vi "Main.vi"   [LabVIEW 2020]
uses:
  Controls/Application Event Message.ctl
  Controls/Application Events.ctl
  Controls/Application Modules.ctl
  Controls/Module Message.ctl
  Error/Controls/Error Message.ctl
  Controls/Module Operational Loop Data.ctl
  Controls/Module State.ctl
types:
  T1 = typedef "Application Events.ctl" = enum16{"Initialize", "Shutdown", "UI: Login", "UI: Withdrawal", "UI: Terminate", "UI: Fast Cash", "UI: Balance Inquiry", "UI: Deposit", "UI: New Transaction", "UI: Card Reader", "UI: On Account Number", "UI: Transaction Timeout", "Controller: Idle", "Controller: Invalid Login", "Controller: Broadcast Balance "}
  T2 = typedef "Module State.ctl" = enum16{"Initial", "Idle", "Login", "Balance Inquiry", "Deposit", "Withdrawal", "Fast Cash", "Terminate"}
  T3 = typedef "Module Operational Loop Data.ctl" = cluster{"State":T2}
  T4 = typedef "Error Message.ctl" = cluster{"Source":T5, "Event":T1, "Error To Handle":errorcluster}
  T5 = typedef "Application Modules.ctl" = enum16{"Controller", "User Console", "Display Console", "Error Handler", "Database Module"}
  T6 = typedef "Module Message.ctl" = cluster{"Source":T5, "Event":T1, "Data":variant}
  T7 = typedef "Application Event Message.ctl" = cluster{"Source":T5, "Event":T1, "Data":variant}
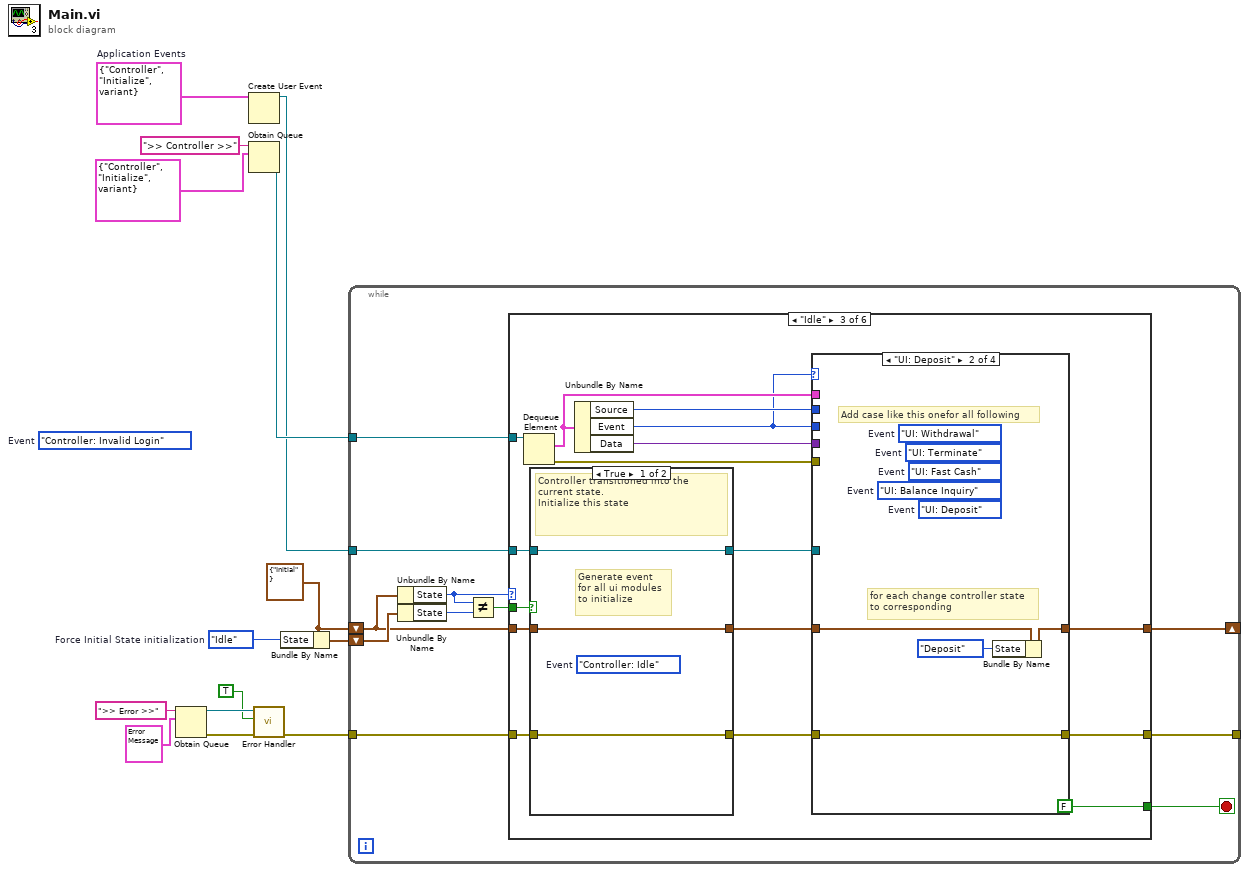
[diagram p0: block diagram]
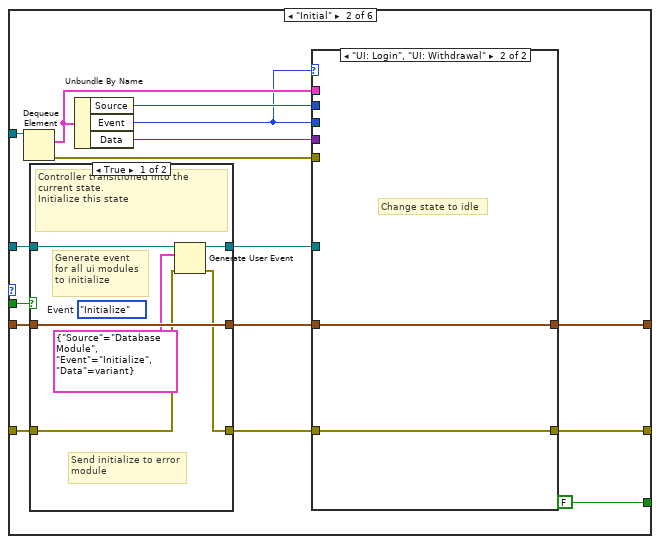
[diagram p3: hidden frame]
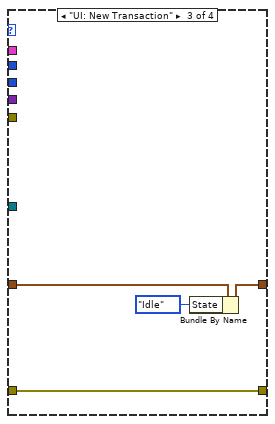
[diagram p7: hidden frame]
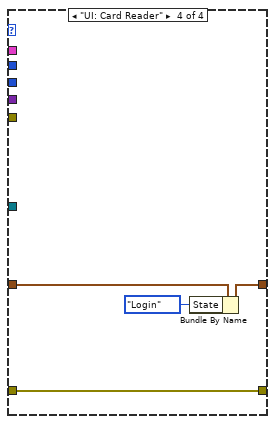
[diagram p8: hidden frame]
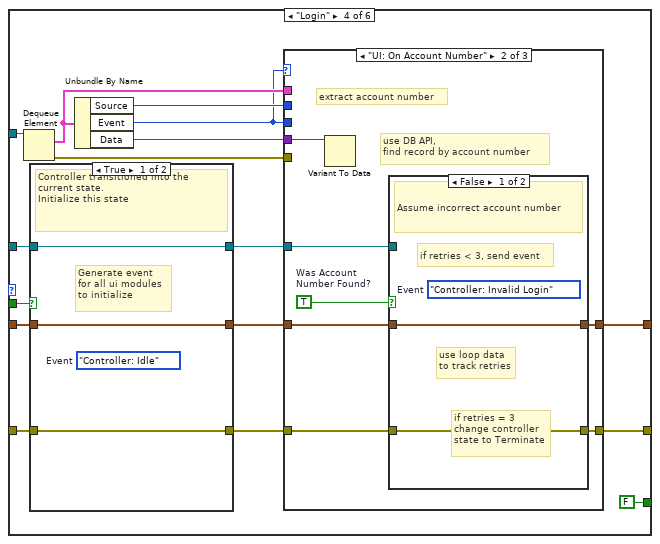
[diagram p10: hidden frame]
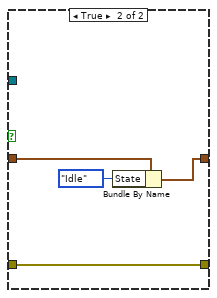
[diagram p12: hidden frame]
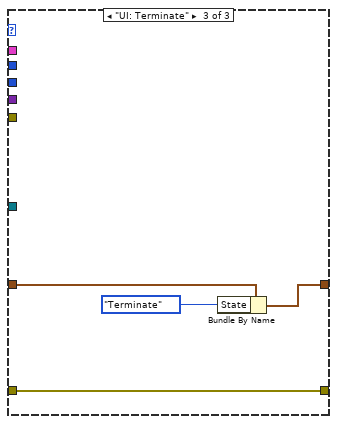
[diagram p13: hidden frame]
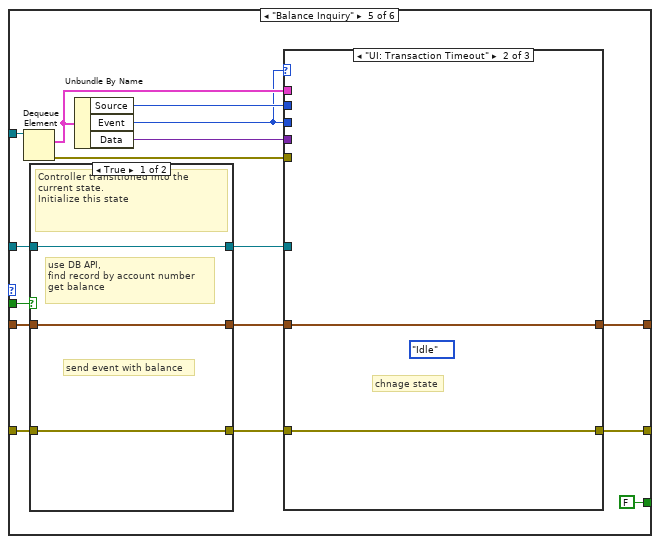
[diagram p15: hidden frame]
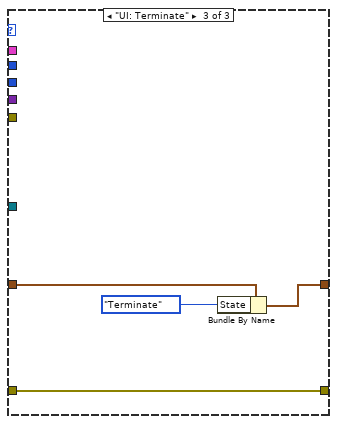
[diagram p17: hidden frame]
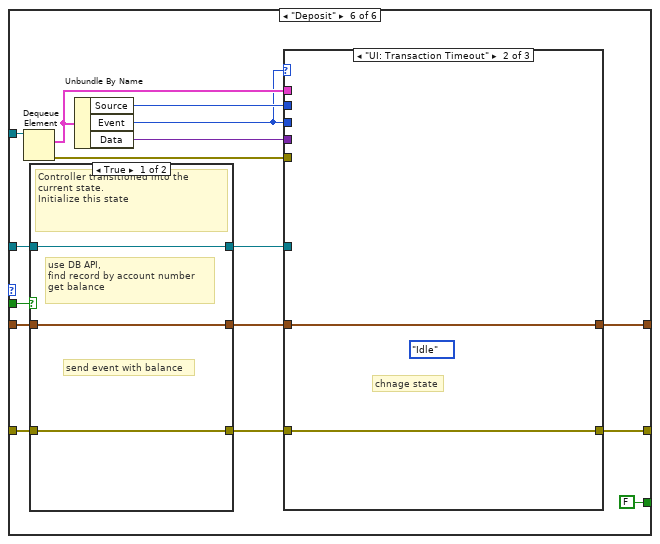
[diagram p19: hidden frame]
diagram:
  (unwired) Application_Events."Controller: Invalid Login"  # Event
  w1 = Module_State."Idle"  # Force Initial State initialization
  w3 = T3 {"State"=enum."Initial"}
  w14 = T7 {"Source"=enum."Controller", "Event"=enum."Initialize", "Data"=variant}  # Application Events
  n1 = Obtain Queue(name (unnamed)=">> Error >>", element data type=T4 {"Source"=enum."Controller", "Event"=enum."Initialize", "Error To Handle"={"status"=FALSE, "code"=0, "source"=""}}) -> (queue out=w8:refnum<queue>, error out=w9:errorcluster)  [unwired: 3 in, 1 out]
  n2 = Create User Event(user event datatype=w14) -> (user event=w4:refnum<user-event>)  [unwired: 1 in, 1 out]
  n3 = Obtain Queue(name (unnamed)=">> Controller >>", element data type=T6 {"Source"=enum."Controller", "Event"=enum."Initialize", "Data"=variant}) -> (queue out=w5:refnum<queue>)  [unwired: 3 in, 2 out]
  n4 = call "Error Handler.vi"("error in"=w9, "Load Reference?"=TRUE, "Error Queue"=w8) -> ("error out"=w6:errorcluster)  [unwired: 8 in]
  n5 = Bundle By Name(cluster=w3, "State"=w1) -> (w2:T3)
  n6 = while {
    tunnel: w6 -> [w17]
    shift-right: [w25] -> _
    shift-left: w3 -> [w23]
    shift-left: w2 -> [w24]
    tunnel: w5 -> [w18]
    tunnel: [w16] -> _
    tunnel: w4 -> [w15]
    stop <- w20 stop-if-true
    n7 = Unbundle By Name(w23) -> ("State"=w21:T2)
    n8 = Unbundle By Name(w24) -> ("State"=w22:T2)
    n9 = Not Equal?(x=w21, y=w22) -> (x != y?=w19:bool)
    n10 = case shown="\"Idle\"" w21 {
      tunnel: [w27 w36 w65 w101 w142 w172] -> w25
      tunnel: w23 -> [w27 w42 w71 w107 w148 w178]
      tunnel: [_ FALSE FALSE FALSE FALSE FALSE] -> w20
      tunnel: w19 -> [_ w41 w70 w106 w147 w177]
      tunnel: w18 -> [_ w40 w69 w105 w146 w176]
      tunnel: [w26 w38 w67 w103 w144 w174] -> w16
      tunnel: w17 -> [w26 w39 w68 w104 w145 w175]
      tunnel: w15 -> [_ w28 w57 w93 w134 w164]
      frame Default {
      }
      frame "Initial" {
        n11 = Dequeue Element(queue=w40) -> (element=w34:T6, error out=w30:errorcluster)  [unwired: 2 in, 2 out]
        n12 = case shown="True" w41 {
          tunnel: [w53 w56] -> w35
          tunnel: w42 -> [w53 w56]
          tunnel: [w50 w55] -> w37
          tunnel: w39 -> [w51 w55]
          tunnel: [w49 w54] -> w29
          tunnel: w28 -> [w52 w54]
          frame True {
            (unwired) Application_Events."Initialize"  # Event
            # "Send initialize to error\nmodule"
            # "Generate event\nfor all ui modules\nto initialize"
            # "Controller transitioned into the current state.\nInitialize this state"
            n13 = Generate User Event(user event=w52, event data cluster=T7 {"Source"=enum."Database Module", "Event"=enum."Initialize", "Data"=variant} ("event data"), error in=w51) -> (user event out=w49:refnum<user-event>, error out=w50:errorcluster)  [unwired: 1 in]
          }
          frame False {
            # "No State transisiton detected"
          }
        }
        n14 = Unbundle By Name(w34) -> ("Source"=w33:T5, "Event"=w31:T1, "Data"=w32:variant)
        n15 = case shown="\"UI: Login\", \"UI: Withdrawal\"" w31 {
          tunnel: [w45 w47] -> w38
          tunnel: w37 -> [w45 w47]
          tunnel: [w44 w46] -> w36
          tunnel: w35 -> [w44 w46]
          tunnel: w34 -> [_ _]
          tunnel: w33 -> [_ _]
          tunnel: w31 -> [_ _]
          tunnel: w32 -> [_ _]
          tunnel: w30 -> [_ _]
          tunnel: w29 -> [_ _]
          frame Default {
          }
          frame "UI: Login", "UI: Withdrawal" {
            # "Change state to idle"
          }
        }
      }
      frame "Idle" {
        n16 = Dequeue Element(queue=w69) -> (element=w63:T6, error out=w59:errorcluster)  [unwired: 2 in, 2 out]
        n17 = case shown="True" w70 {
          tunnel: [w89 w92] -> w64
          tunnel: w71 -> [w89 w92]
          tunnel: [w88 w91] -> w66
          tunnel: w68 -> [w88 w91]
          tunnel: [w87 w90] -> w58
          tunnel: w57 -> [w87 w90]
          frame True {
            (unwired) Application_Events."Controller: Idle"  # Event
            # "Generate event\nfor all ui modules\nto initialize"
            # "Controller transitioned into the current state.\nInitialize this state"
          }
          frame False {
            # "No State transisiton detected"
          }
        }
        n18 = Unbundle By Name(w63) -> ("Source"=w62:T5, "Event"=w60:T1, "Data"=w61:variant)
        n19 = case shown="\"UI: Deposit\"" w60 {
          tunnel: [w74 w78 w82 w86] -> w67
          tunnel: w66 -> [w74 w78 w82 w86]
          tunnel: [w73 w75 w79 w83] -> w65
          tunnel: w64 -> [w73 w77 w81 w85]
          tunnel: w63 -> [_ _ _ _]
          tunnel: w62 -> [_ _ _ _]
          tunnel: w60 -> [_ _ _ _]
          tunnel: w61 -> [_ _ _ _]
          tunnel: w59 -> [_ _ _ _]
          tunnel: w58 -> [_ _ _ _]
          frame Default {
          }
          frame "UI: Deposit" {
            (unwired) Application_Events."UI: Deposit"  # Event
            (unwired) Application_Events."UI: Balance Inquiry"  # Event
            (unwired) Application_Events."UI: Fast Cash"  # Event
            (unwired) Application_Events."UI: Terminate"  # Event
            (unwired) Application_Events."UI: Withdrawal"  # Event
            # "for each change controller state\nto corresponding"
            # "Add case like this onefor all following"
            n20 = Bundle By Name(cluster=w77, "State"=Module_State."Deposit") -> (w75:T3)
          }
          frame "UI: New Transaction" {
            n21 = Bundle By Name(cluster=w81, "State"=Module_State."Idle") -> (w79:T3)
          }
          frame "UI: Card Reader" {
            n22 = Bundle By Name(cluster=w85, "State"=Module_State."Login") -> (w83:T3)
          }
        }
      }
      frame "Login" {
        n23 = Dequeue Element(queue=w105) -> (element=w99:T6, error out=w95:errorcluster)  [unwired: 2 in, 2 out]
        n24 = case shown="True" w106 {
          tunnel: [w130 w133] -> w100
          tunnel: w107 -> [w130 w133]
          tunnel: [w129 w132] -> w102
          tunnel: w104 -> [w129 w132]
          tunnel: [w128 w131] -> w94
          tunnel: w93 -> [w128 w131]
          frame True {
            (unwired) Application_Events."Controller: Idle"  # Event
            # "Generate event\nfor all ui modules\nto initialize"
            # "Controller transitioned into the current state.\nInitialize this state"
          }
          frame False {
            # "No State transisiton detected"
          }
        }
        n25 = Unbundle By Name(w99) -> ("Source"=w98:T5, "Event"=w96:T1, "Data"=w97:variant)
        n26 = case shown="\"UI: On Account Number\"" w96 {
          tunnel: [w110 w113 w127] -> w103
          tunnel: w102 -> [w110 w112 w127]
          tunnel: [w109 w116 w124] -> w101
          tunnel: w100 -> [w109 w117 w126]
          tunnel: w99 -> [_ _ _]
          tunnel: w98 -> [_ _ _]
          tunnel: w96 -> [_ _ _]
          tunnel: w97 -> [_ w115 _]
          tunnel: w95 -> [_ _ _]
          tunnel: w94 -> [_ w111 _]
          frame Default {
          }
          frame "UI: On Account Number" {
            w114 = TRUE  # Was Account  Number Found?
            # "use DB API,\nfind record by account number"
            # "extract account number"
            n27 = Variant To Data(Variant=w115) -> ()  [unwired: 2 in, 2 out]
            n28 = case shown="False" w114 {
              tunnel: w117 -> [w119 w123]
              tunnel: [w119 w121] -> w116
              tunnel: [w118 w120] -> w113
              tunnel: w112 -> [w118 w120]
              tunnel: w111 -> [_ _]
              frame False {
                (unwired) Application_Events."Controller: Invalid Login"  # Event
                # "if retries < 3, send event"
                # "if retries = 3\nchange controller\nstate to Terminate"
                # "use loop data\nto track retries"
                # "Assume incorrect account number"
              }
              frame True {
                n29 = Bundle By Name(cluster=w123, "State"=Module_State."Idle") -> (w121:T3)
              }
            }
          }
          frame "UI: Terminate" {
            n30 = Bundle By Name(cluster=w126, "State"=Module_State."Terminate") -> (w124:T3)
          }
        }
      }
      frame "Balance Inquiry" {
        n31 = Dequeue Element(queue=w146) -> (element=w140:T6, error out=w136:errorcluster)  [unwired: 2 in, 2 out]
        n32 = case shown="True" w147 {
          tunnel: [w160 w163] -> w141
          tunnel: w148 -> [w160 w163]
          tunnel: [w159 w162] -> w143
          tunnel: w145 -> [w159 w162]
          tunnel: [w158 w161] -> w135
          tunnel: w134 -> [w158 w161]
          frame True {
            # "send event with balance"
            # "use DB API,\nfind record by account number\nget balance"
            # "Controller transitioned into the current state.\nInitialize this state"
          }
          frame False {
            # "No State transisiton detected"
          }
        }
        n33 = Unbundle By Name(w140) -> ("Source"=w139:T5, "Event"=w137:T1, "Data"=w138:variant)
        n34 = case shown="\"UI: Transaction Timeout\"" w137 {
          tunnel: [w151 w152 w157] -> w144
          tunnel: w143 -> [w151 w152 w157]
          tunnel: [w150 w153 w154] -> w142
          tunnel: w141 -> [w150 w153 w156]
          tunnel: w140 -> [_ _ _]
          tunnel: w139 -> [_ _ _]
          tunnel: w137 -> [_ _ _]
          tunnel: w138 -> [_ _ _]
          tunnel: w136 -> [_ _ _]
          tunnel: w135 -> [_ _ _]
          frame Default {
          }
          frame "UI: Transaction Timeout" {
            (unwired) Module_State."Idle" ("State")
            # "chnage state"
          }
          frame "UI: Terminate" {
            n35 = Bundle By Name(cluster=w156, "State"=Module_State."Terminate") -> (w154:T3)
          }
        }
      }
      frame "Deposit" {
        n36 = Dequeue Element(queue=w176) -> (element=w170:T6, error out=w166:errorcluster)  [unwired: 2 in, 2 out]
        n37 = case shown="True" w177 {
          tunnel: [w190 w193] -> w171
          tunnel: w178 -> [w190 w193]
          tunnel: [w189 w192] -> w173
          tunnel: w175 -> [w189 w192]
          tunnel: [w188 w191] -> w165
          tunnel: w164 -> [w188 w191]
          frame True {
            # "send event with balance"
            # "use DB API,\nfind record by account number\nget balance"
            # "Controller transitioned into the current state.\nInitialize this state"
          }
          frame False {
            # "No State transisiton detected"
          }
        }
        n38 = Unbundle By Name(w170) -> ("Source"=w169:T5, "Event"=w167:T1, "Data"=w168:variant)
        n39 = case shown="\"UI: Transaction Timeout\"" w167 {
          tunnel: [w181 w182 w187] -> w174
          tunnel: w173 -> [w181 w182 w187]
          tunnel: [w180 w183 w184] -> w172
          tunnel: w171 -> [w180 w183 w186]
          tunnel: w170 -> [_ _ _]
          tunnel: w169 -> [_ _ _]
          tunnel: w167 -> [_ _ _]
          tunnel: w168 -> [_ _ _]
          tunnel: w166 -> [_ _ _]
          tunnel: w165 -> [_ _ _]
          frame Default {
          }
          frame "UI: Transaction Timeout" {
            (unwired) Module_State."Idle" ("State")
            # "chnage state"
          }
          frame "UI: Terminate" {
            n40 = Bundle By Name(cluster=w186, "State"=Module_State."Terminate") -> (w184:T3)
          }
        }
      }
    }
  }
